vi "Utest4.vi"() -> ()   [LabVIEW 2010]
uses:
  Instance           2 14Saved   Utest4 .vi
  Instance           3 14Saved   Utest4 .vi
  Instance           5 14Saved   Utest4 .vi
  Instance           4 14Saved   Utest4 .vi
  user32.dll
panel:
  in  "Case Constant\n(See Context Help)":bool
  out "concatenated string":string
  out "return code":i32
  out "standard error":string
  out "error out":errorcluster
  out "standard output":string
  out "Boolean":bool
  in  "OK Button":bool
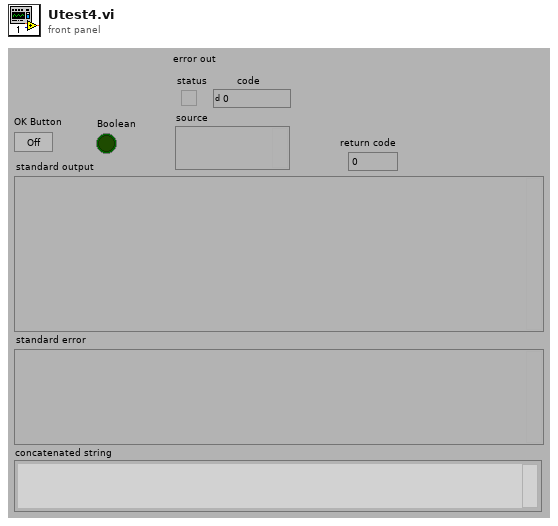
[diagram p1: front panel]
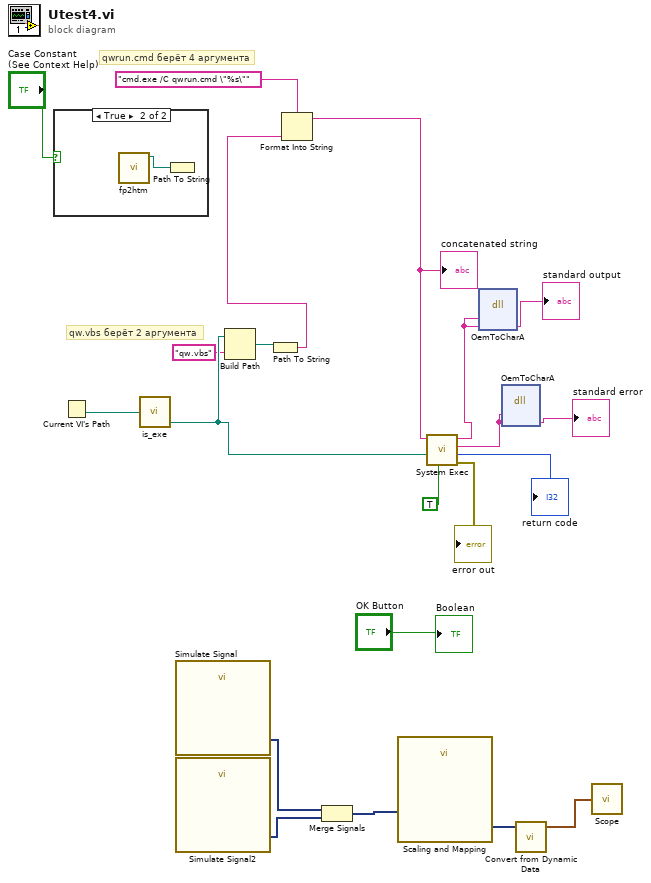
[diagram p0: block diagram]
diagram:
  # "qw.vbs берёт 2 аргумента"
  # "qwrun.cmd берёт 4 аргумента"
  n1 = case shown="True" "Case Constant\n(See Context Help)" {
    frame False {
    }
    frame True {
      n2 = call "fp2htm.vi"() -> ("path"=w22:path)  [unwired: 7 in]
      n3 = Path To String(path=w22) -> ()  [unwired: 1 out]
    }
  }
  n4 = Current VI's Path() -> (path=w13:path)
  n5 = call "is_exe.vi"("path"=w13) -> ("actual path"=w7:path)  [unwired: 2 in, 2 out]
  n6 = call "Simulate Signal"() -> ("Sine"=w21:dynamicdata)  [unwired: 14 in, 1 out]
  n7 = call "Simulate Signal2"() -> ("Triangle"=w20:dynamicdata)  [unwired: 14 in, 1 out]
  n8 = Build Path(base path=w7, name or relative path="qw.vbs") -> (appended path=w5:path)
  n9 = Path To String(path=w5) -> (string=w3:string)
  n10 = Format Into String(format string="cmd.exe /C qwrun.cmd \"%s\"" ("command line"), w3) -> (resulting string=w2:string)  [unwired: 2 in, 1 out]
  "concatenated string" <- w2
  n11 = Merge Signals(w21, w20) -> (w18:dynamicdata)
  n12 = call "Scaling and Mapping"("Signals"=w18) -> ("Scaled Signals"=w17:dynamicdata)  [unwired: 9 in, 1 out]
  n13 = call <vilib>:"System Exec.vi"("run minimized? (F)"=TRUE, "working directory"=w7, "command line"=w2) -> ("error out"=→"error out":errorcluster, "return code"=→"return code":i32, "standard error"=w11:string, "standard output"=w9:string)  [unwired: 5 in]
  n14 = dll-call lib="user32.dll" fn="OemToCharA"(w9, w9) -> (→"standard output":string)  [unwired: 5 in, 2 out]
  n15 = dll-call lib="user32.dll" fn="OemToCharA"(w11, w11) -> (→"standard error":string)  [unwired: 5 in, 2 out]
  n16 = call "Convert from Dynamic Data"("Dynamic Data Type"=w17) -> ("Array of Waveform"=w19:waveform(dbl)[])  [unwired: 3 in]
  n17 = call "Scope.vi"("Array"=w19) -> ()
  "Boolean" <- "OK Button"
